vi "LoadPortCValues.vi"(8 "error in (no error)":errorcluster) -> (0 "error out":errorcluster)   [LabVIEW 2015]
uses:
  Drive/Implementation/Advanced Drive VIs/PID Type Def.ctl
  Port/PortC Settings Type Def.ctl
  Detailed Motor Type Def.ctl
  <vilib>/Rock Robotics/WPI/MotorControl/WPI_MotorControlDeviceRef.ctl
  <vilib>/Rock Robotics/WPI/MotorControl/WPI_MotorControlType.ctl
  <vilib>/Rock Robotics/SystemInterfaces/DIO/FPGA_DIOPWMChannel.ctl
  <vilib>/Rock Robotics/WPI/PWM/WPI_PWMDeadband.ctl
  <vilib>/Rock Robotics/WPI/CAN/Jaguar/SubVIs/WPI_CANJaguar_ControlMode.ctl
  <vilib>/Rock Robotics/WPI/CAN/TalonSRX/WPI_CANTalonSRX_APIControlMode.ctl
  <vilib>/Rock Robotics/Network Tables/NT Read Numeric Array.vi
  Port/PortC Global.vi
  Robot Global Data.vi
panel:
  out "Settings":T1={"Down"=-230.0, "Up"=140.0, "Increments"=-230.0, "Final Pos"=-230.0}
  out "PID":T2
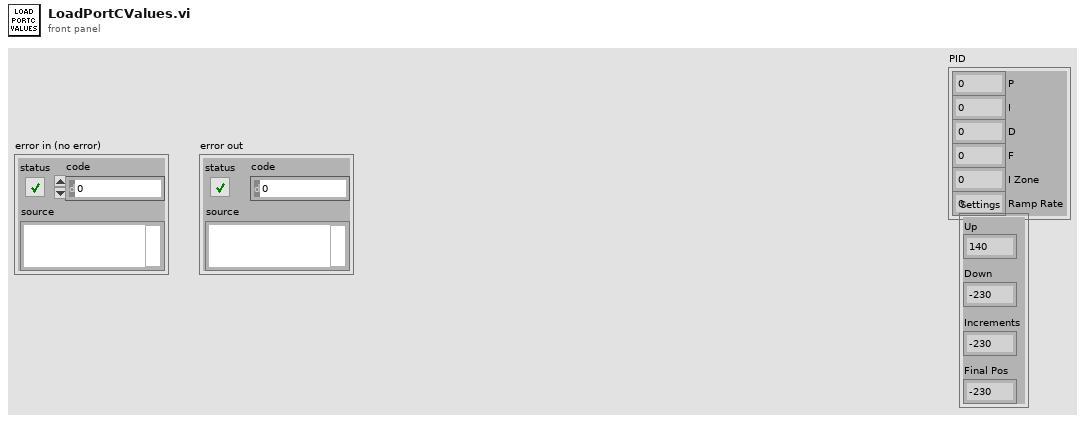
[diagram p1: front panel]
types:
  T1 = typedef "PortC Settings Type Def.ctl" = cluster{"Down":dbl, "Up":dbl, "Increments":dbl, "Final Pos":dbl}
  T2 = typedef "PID Type Def.ctl" = cluster{"P":dbl, "I":dbl, "D":dbl, "F":dbl, "I Zone":dbl, "Ramp Rate":dbl}
  T3 = typedef "Detailed Motor Type Def.ctl" = cluster{"MotorRef":T4, "Encoder Ticks Per Rev":dbl, "Set Position":dbl, "Wheel Radius":dbl}
  T4 = typedef "WPI_MotorControlDeviceRef.ctl" = cluster{"DeviceStatus":errorcluster, "Type":T5, "PWM":cluster{"PWM Channel":T6, "DeadBand":T7}, "CAN":cluster{"Device Number":u8, "Control Mode":T8, "Semaphore":T9, "Max Vout":dbl, "TalonSRX Control Mode":T10}, "Invert":bool}
  T5 = typedef "WPI_MotorControlType.ctl" = enum16{"PWM", "CAN", "CANTalonSRX"}
  T6 = typedef "FPGA_DIOPWMChannel.ctl" = enum8{"PWM 0", "PWM 1", "PWM 2", "PWM 3", "PWM 4", "PWM 5", "PWM 6", "PWM 7", "PWM 8", "PWM 9", "PWM MXP 0", "PWM MXP 1", "PWM MXP 2", "PWM MXP 3", "PWM MXP 4", "PWM MXP 5", "PWM MXP 6", "PWM MXP 7", "PWM MXP 8", "PWM MXP 9", "Invalid"}
  T7 = typedef "WPI_PWMDeadband.ctl" = cluster{"Name":string, "maxPositivePwm":i32, "minPositivePwm":i32, "centerPwm":i32, "maxNegativePwm":i32, "minNegativePwm":i32, "angularRange":u16}
  T8 = typedef "WPI_CANJaguar_ControlMode.ctl" = enum8{"Percent VBus", "Current", "Speed", "Position", "Voltage"}
  T9 = typedef "Semaphore RefNum" = refnum<k1>
  T10 = typedef "WPI_CANTalonSRX_APIControlMode.ctl" = enum8{"Percent VBus", "Speed", "Position", "Slave", "Unchanged / Invalid", "Voltage Compensation", "Current", "Motion Profile"}
  T11 = typedef "WPI_CANTalonSRX_GlobalStatus.ctl" = cluster{"Applied Throttle":dbl, "Module Enabled":bool, "CAN Error":errorcluster, "Closed Loop Error":dbl, "Forward Limit Switch Closed":bool, "Reverse Limit Switch Closed":bool, "Sensor Position":dbl, "Sensor Velocity":dbl, "Current":dbl, "Sticky Fault - Over Temp":bool, "Sticky Fault - Under Voltage":bool, "Sticky Fault - Forward Limit":bool, "Sticky Fault - Reverse Limit":bool, "Sticky Fault - Forward Soft Limit":bool, "Sticky Fault - Reverse Soft Limit":bool, "Brake is Enabled":bool, "Encoder Position":dbl, "Encoder Velocity":dbl, "Encoder Index Count":dbl, "Encoder A Pin State":bool, "Encoder B Pin State":bool, "Encoder Index Pin State":bool, "Analog In":dbl, "Analog In Velocity":dbl, "Temperature (C)":dbl, "Battery Voltage":dbl, "Control 5 Is Supported":bool, "Current Profile Slot Select":dbl, "Pos Div 8":bool, "Vel Div 4":bool, "Pulse Width Position":i32, "Pulse Width Velocity":i32, "Pulse Width Rise To Rise (us)":i32, "Pulse Width Rise To Fall (us)":i32, "Mot Prof Active Is Under Run":bool, "Mot Prof Active Has Under Run":bool, "Mot Prof Active Is Last":bool, "Mot Prof Active Velocity Only":bool, "Mot Prof Active Is Valid":bool, "Mot Prof Buffer Is Full":bool, "Mot Prof Active Profile Slot Select":i32, "Mot Prof NextID":i32, "Mot Prof Count":i32, "Mot Prof Active Velocity":dbl, "Mot Prof Active Position":dbl, "Mot Prof Output Enable":i32}
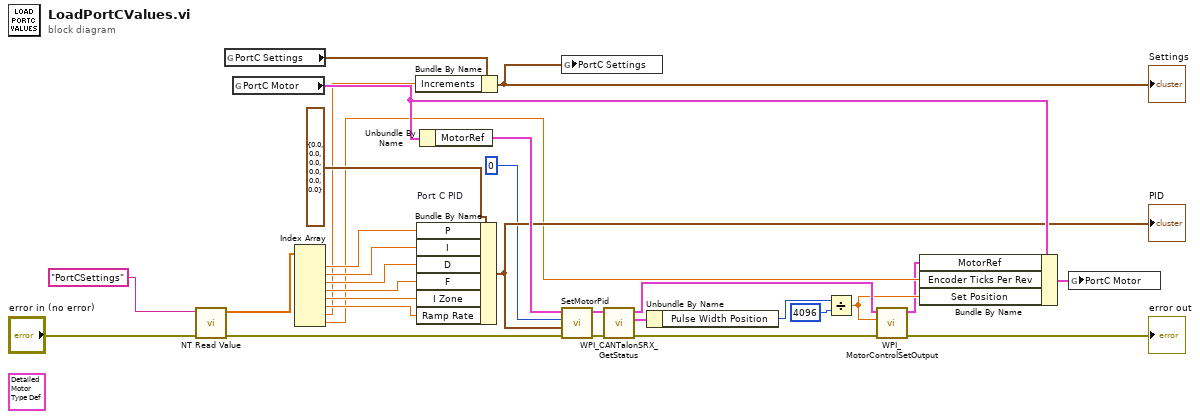
[diagram p0: block diagram]
diagram:
  (unwired) T3 {"MotorRef"={"DeviceStatus"={"status"=FALSE, "code"=0, "source"=""}, "Type"=enum."PWM", "PWM"={"PWM Channel"=enum."Invalid", "DeadBand"={"Name"="", "maxPositivePwm"=0, "minPositivePwm"=0, "centerPwm"=0, "maxNegativePwm"=0, "minNegativePwm"=0, "angularRange"=0}}, "CAN"={"Device Number"=0, "Control Mode"=enum."Percent VBus", "Semaphore"=refnum, "Max Vout"=12.0, "TalonSRX Control Mode"=enum."Percent VBus"}, "Invert"=FALSE}, "Encoder Ticks Per Rev"=0.0, "Set Position"=0.0, "Wheel Radius"=0.0} ("Detaled Motor Type Def")
  n1 = call-poly <vilib>:"NT Read Value.vi"("error in"="error in (no error)", "Name"="PortCSettings") -> ("error out"=w14:errorcluster, "Numeric Array"=w19:dbl[])  [unwired: 8 in]
  n2 = global read "Robot Global Data.vi" "PortC Settings"() -> (w29:T1)
  n3 = global read "PortC Global.vi" "PortC Motor"() -> (w27:T3)
  n4 = Index Array(array=w19) -> (element #1=w20:dbl, element #2=w21:dbl, element #3=w22:dbl, element #4=w23:dbl, element #5=w24:dbl, element #6=w25:dbl, element #7=w11:dbl, element #8=w12:dbl)  [unwired: 8 in]
  n5 = Bundle By Name(cluster=w29, "Increments"=w11) -> (w13:T1)
  "Settings" <- w13
  n6 = Bundle By Name "Port C PID"(cluster=T2 {"P"=0.0, "I"=0.0, "D"=0.0, "F"=0.0, "I Zone"=0.0, "Ramp Rate"=0.0} ("PID"), "P"=w20, "I"=w21, "D"=w22, "F"=w23, "I Zone"=w24, "Ramp Rate"=w25) -> (w26:T2)
  "PID" <- w26
  n7 = Unbundle By Name(w27) -> ("MotorRef"=w30:T4)
  n8 = global write "Robot Global Data.vi" "PortC Settings"(w13) -> ()
  n9 = call "SetMotorPid.vi"("error in (no error)"=w14, "PID"=w26, "Parameter Slot"=u8 0, "Motor Ref In"=w30) -> ("error out"=w4:errorcluster, "Motor Ref Out"=w3:T4)  [unwired: 6 in]
  n10 = call <vilib>:"WPI_CANTalonSRX_GetStatus.vi"("error in (no error)"=w4, "CAN Talon SRX Ref"=w3) -> ("error out"=w8:errorcluster, "Talon SRX Status"=w7:T11, "CAN Talon SRX Ref"=w10:T4)  [unwired: 7 in]
  n11 = Unbundle By Name(w7) -> ("Pulse Width Position"=w6:i32)
  n12 = Divide(x=w6, y=4096) -> (x/y=w5:dbl)
  n13 = call <vilib>:"WPI_MotorControlSetOutput.vi"("error in (no error)"=w8, "Output"=w5, "MotorControlDevRef"=w10) -> ("error out"=→"error out":errorcluster, "MotorControlDevRef"=w2:T4)  [unwired: 6 in, 1 out]
  n14 = Bundle By Name(cluster=w27, "MotorRef"=w2, "Encoder Ticks Per Rev"=w12, "Set Position"=w5) -> (w28:T3)
  n15 = global write "PortC Global.vi" "PortC Motor"(w28) -> ()
